vi "CU_testMahalanobis.vi"(6 "DataTypes":T1=enum."Test Data", 7 "Indices":i8[](array[numeric]), 8 "error in":errorcluster, 9 "Mean vectors":dbl[][](array[numeric]), 10 "Covariance matricies":dbl[][][](array[numeric]), 11 "ClassifierClass in":refnum<class "ClassifierClass.lvclass">) -> (0 "error out":errorcluster, 1 "Confusion Matrix":i32[][](array[numeric]), 2 "Accuracy":dbl, 3 "ClassifierClass out":refnum<class "ClassifierClass.lvclass">)   [LabVIEW 2016, in "Classifier.lvlib" / "ClassifierClass.lvclass"]
uses:
  ClassifierClass.lvclass
  CU_DataTypes.ctl
  ClassifierClass.lvclass/ClassifierClass.ctl
  <vilib>/Analysis/baseanly.llb/Vector x A.vi
  <vilib>/Analysis/baseanly.llb/Real Dot Product.vi
  CU_CohenKappa.vi
  <vilib>/addons/Machine Learning/NILabs_MLT.lvlib
  <vilib>/Analysis/NI_AALBase.lvlib
  Classifier.lvlib
panel:
  # "This VI is a part of BCI Design library, http://www.ru-bci.org \nCopyright © 2020, Sotnikov Peter, All rights reserved. License: CC BY-NC 4.0"
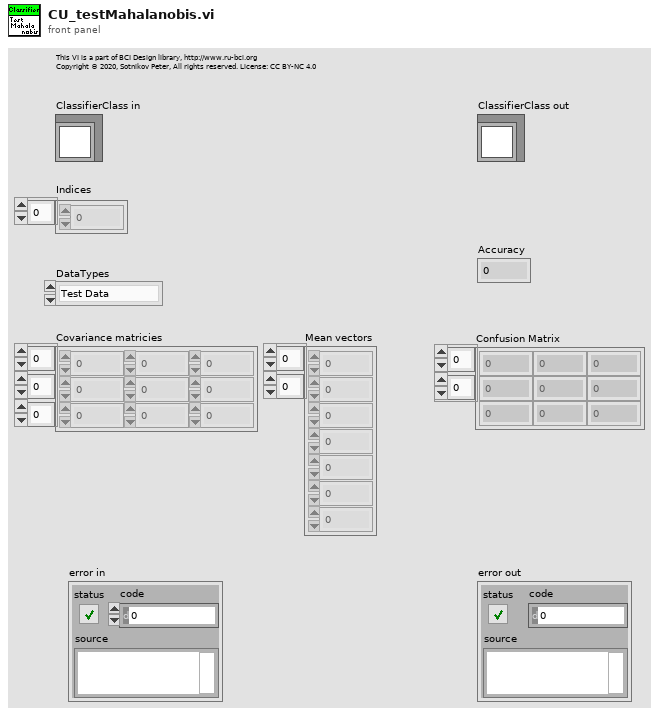
[diagram p1: front panel]
types:
  T1 = typedef "Classifier.lvlib/CU_DataTypes.ctl" = enum16{"Training Data", "Test Data", "Training Data (cross-check)", "Test Data (cross-check)"}
  T2 = typedef "XML_EEG_Features.lvlib/XML_FF_Trial.ctl" = cluster{"ClassLabel":string, "FeatureVector":dbl[]}
  T3 = typedef "Classifier.lvlib/CU_ClassifierQualityMeasure.ctl" = enum16{"Accuracy", "Cohen's kappa"}
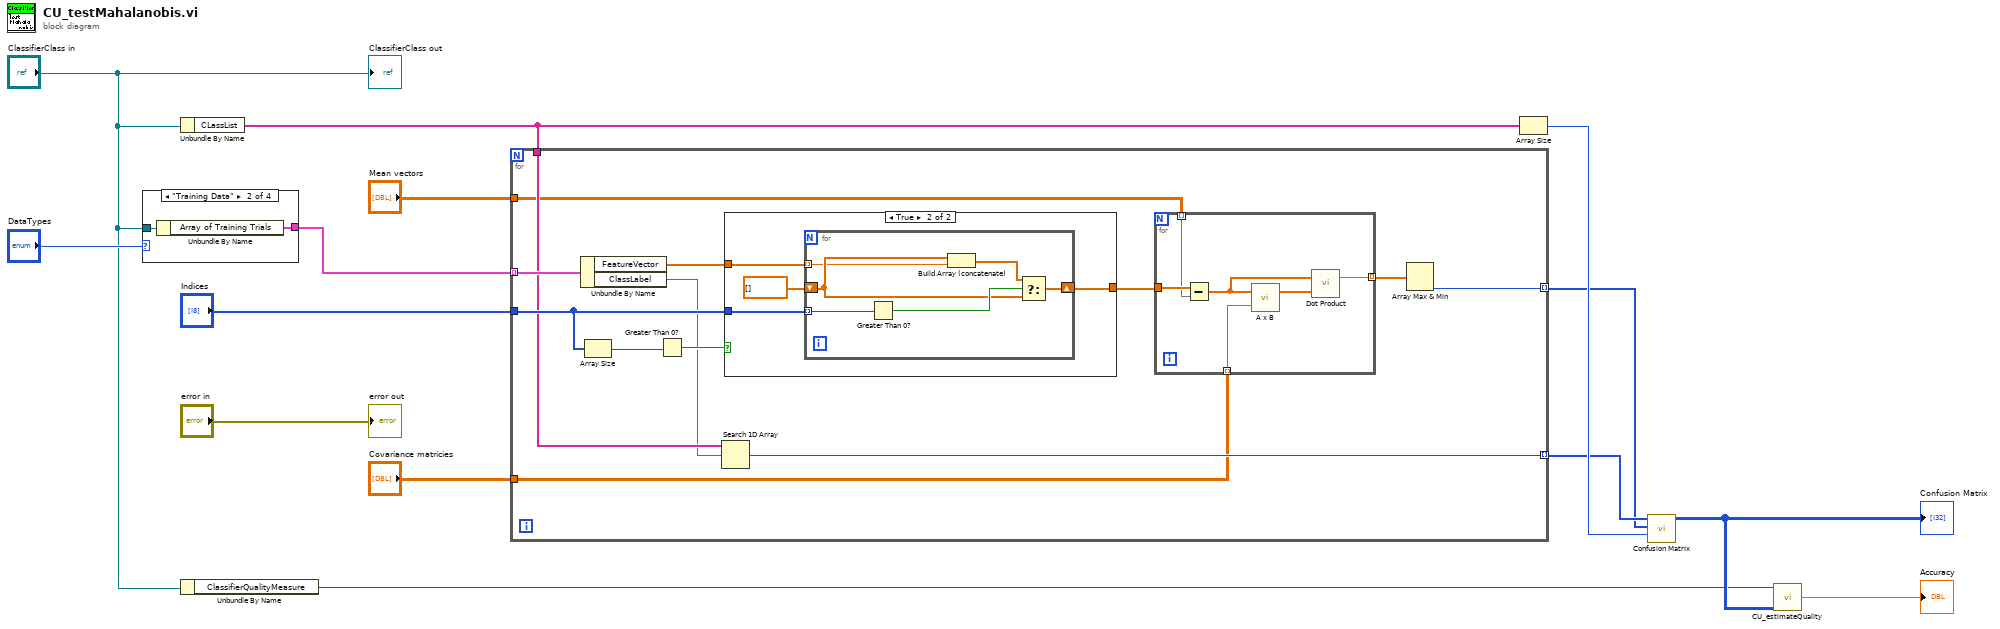
[diagram p0: block diagram]
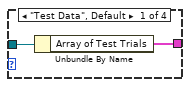
[diagram p2: hidden frame]
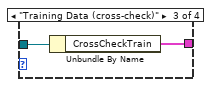
[diagram p3: hidden frame]
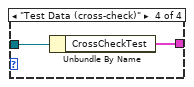
[diagram p4: hidden frame]
diagram:
  n1 = case shown="\"Training Data\"" "DataTypes" {
    tunnel: "ClassifierClass in" -> [w16 w18 w20 w22]
    tunnel: [w15 w17 w19 w21] -> w7
    frame "Test Data", Default {
      n2 = Unbundle By Name(w16) -> ("Array of Test Trials"=w15:T2[])
    }
    frame "Training Data" {
      n3 = Unbundle By Name(w18) -> ("Array of Training Trials"=w17:T2[])
    }
    frame "Training Data (cross-check)" {
      n4 = Unbundle By Name(w20) -> ("CrossCheckTrain"=w19:T2[])
    }
    frame "Test Data (cross-check)" {
      n5 = Unbundle By Name(w22) -> ("CrossCheckTest"=w21:T2[])
    }
  }
  n6 = Unbundle By Name("ClassifierClass in") -> ("CLassList"=w13:string[])
  n7 = Unbundle By Name("ClassifierClass in") -> ("ClassifierQualityMeasure"=w2:T3)
  n8 = for {
    tunnel: w7 -> [w33] mode=indexing
    tunnel: "Indices" -> [w31]
    tunnel: w13 -> [w30]
    tunnel: [w28] -> w5 mode=indexing
    tunnel: [w23] -> w4 mode=indexing
    tunnel: "Mean vectors" -> [w26]
    tunnel: "Covariance matricies" -> [w25]
    n9 = Unbundle By Name(w33) -> ("FeatureVector"=w32:dbl[], "ClassLabel"=w29:string)
    n10 = Array Size(array=w31) -> (size(s)=w35:i32)
    n11 = Greater Than 0?(x=w35) -> (x > 0?=w34:bool)
    n12 = Search 1D Array(1D array=w30, element=w29) -> (index of element=w28:i32)  [unwired: 1 in]
    n13 = case shown="True" w34 {
      tunnel: w32 -> [w42 w46]
      tunnel: w31 -> [_ w45]
      tunnel: [w42 w43] -> w27
      frame False {
      }
      frame True {
        n14 = for {
          tunnel: w46 -> [w48] mode=indexing
          tunnel: w45 -> [w52] mode=indexing
          shift-right: [w51] -> w43
          shift-left: dbl[] [] -> [w49]
          n15 = Greater Than 0?(x=w52) -> (x > 0?=w50:bool)
          n16 = Build Array (concatenate)(w49, w48) -> (w47:dbl[])
          n17 = Select(t=w47, s=w50, f=w49) -> (s? t:f=w51:dbl[])
        }
      }
    }
    n18 = for {
      tunnel: w27 -> [w41]
      tunnel: w26 -> [w40] mode=indexing
      tunnel: w25 -> [w39] mode=indexing
      tunnel: [w36] -> w24 mode=indexing
      n19 = Subtract(x=w41, y=w40) -> (x-y=w38:dbl[])
      n20 = call-poly <vilib>:"A x B.vi"("Matrix A"=w39, "Vector V'"=w38) -> ("V' x A"=w37:dbl[])  [unwired: 1 out]
      n21 = call-poly <vilib>:"Dot Product.vi"("Y Vector"=w37, "X Vector"=w38) -> ("X * Y"=w36:dbl)  [unwired: 1 out]
    }
    n22 = Array Max & Min(array=w24) -> (min index (indices)=w23:i32)  [unwired: 3 out]
  }
  n23 = Array Size(array=w13) -> (size(s)=w12:i32)
  n24 = call <vilib>:"Confusion Matrix.vi"("# of classes"=w12, "Predicted class labels"=w4, "Actual class labels"=w5) -> ("Confusion Matrix"=w3:i32[][])  [unwired: 7 in, 1 out]
  "Confusion Matrix" <- w3
  n25 = call "CU_estimateQuality.vi"("Quality Measure in"=w2, "Confusion Matrix in"=w3) -> ("Classification Quality out"=→"Accuracy":dbl)  [unwired: 6 in]
  "error out" <- "error in"
  "ClassifierClass out" <- "ClassifierClass in"
